vi "2 (SubVI).vi"(10 "Scalar":dbl, 11 "Numeric":dbl) -> (3 "Cluster":cluster{dbl[], dbl[]})   [LabVIEW 2020]
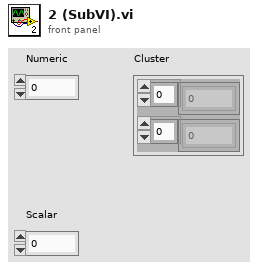
[diagram p1: front panel]
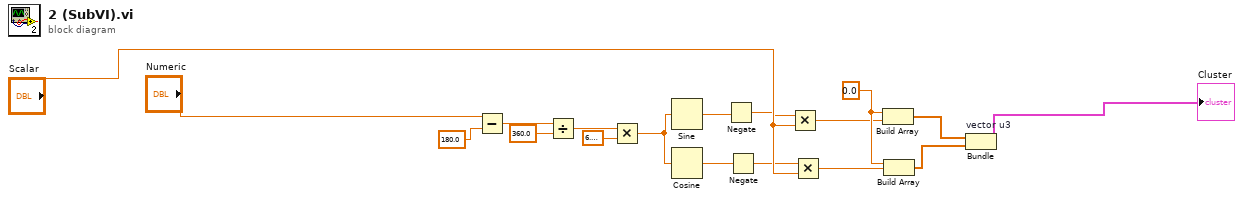
[diagram p0: block diagram]
diagram:
  w13 = 0.0 ("element")
  n1 = Subtract(x="Numeric", y=180.0) -> (x-y=w2:dbl)
  n2 = Divide(x=w2, y=360.0) -> (x/y=w4:dbl)
  n3 = Multiply(x=w4, y=6.283185307179586) -> (x*y=w6:dbl)
  n4 = Sine(x=w6) -> (sin(x)=w7:dbl)
  n5 = Cosine(x=w6) -> (cos(x)=w8:dbl)
  n6 = Negate(x=w7) -> (-x=w10:dbl)
  n7 = Negate(x=w8) -> (-x=w9:dbl)
  n8 = Multiply(x=w10, y="Scalar") -> (x*y=w12:dbl)
  n9 = Multiply(x=w9, y="Scalar") -> (x*y=w11:dbl)
  n10 = Build Array(w13, w12) -> (w14:dbl[])
  n11 = Build Array(w13, w11) -> (w15:dbl[])
  n12 = Bundle "vector u3"(w14, w15) -> (→"Cluster":cluster{dbl[], dbl[]})  [unwired: 1 in]
